vi "player tansition data for all2.vi"() -> ()   [LabVIEW 2013]
panel:
  out "CJ opp ALL":string[][](array[string])
  out "CJ opp left":string[][](array[string])
  out "CJ opp right":string[][](array[string])
  in  "CJ top vs WF":string[][](array[string])=[["3", "36585", "36833", "0 -4 4 -4 0 3 0 4 -4\r\n"], ["3", "37249", "37305", "0 4\r\n"], ["3", "37585", "38105", "1 0 1 -4 1 -4 1 0 2 -2 2 0 -4 0 -2 3 0 -1 1 0 4 -4 1\r\n"], ["3", "38889", "39001", "0 -3 3 0\r\n"], ["3", "39393", "39729", "2 -1 0 4 -1 4 -4 0 -1 1 0 -3 0 -4 1\r\n"], ["3", "40225", "40345", "-4 0 -4 0\r\n"], ["3", "40921", "41041", "-1 0 -1 0 4 0\r\n"], ["3", "41457", "42113", "0 -3 3 0 2 -2 2 0 -3 0 1 0 1 -4 4 -4 1 0 3 -2 0 1 -1 0\r\n"], ["3", "43049", "43241", "0 1 0 2\r\n"], ["3", "43713", "43961", "0 4 -4 1 -4 1 -4 1 -4 0 -3 3 0 2 0 -4\r\n"], ["3", "44425", "44681", "-4 1 0 2 -2 0 -2 3 0 1 0\r\n"], ["3", "45281", "45617", "0 -3 3 0 -1 1 0 -1 0 4 0 -3 4 -4 1 -4 0\r\n"], ["3", "46169", "46585", "0 1 0 3 -3 0 -2 3 -3 0 4 -4 0\r\n"], ["3", "47177", "47593", "0 4 -4 0 -1 0 3 -3 0 -4 0 1 0 -4 4 -4 1\r\n"], ["3", "48425", "49361", "0 1 0 4 -3 0 2 -1 0 4 0 -4 4 -4 0 -4 4 -4 0 4 0 1 0 3 0 -2 3 -2 0 3 -3 0 1 0 4 0 -2\r\n"], ["3", "49961", "50073", "0 1 -1 0\r\n"], ["3", "50529", "50737", "0 -1 0 3 0 -4 4\r\n"], ["3", "52529", "52657", "0 -3 0 -2 2 0 -1 1\r\n"], ["3", "53009", "53137", "0 4 -4 0\r\n"], ["3", "53569", "54641", "0 -3 3 0 3 -3 0 -4 4 -4 0 4 -4 1 0 2 0 -2 3 -2 0 3 0 4 -4 0 2 -2 0 1 -4 4 -4 0 3 0 2 -1 0 1 -4 1 0 3 -2 0 3 0 1\r\n"], ["3", "55161", "55361", "1 0 1 0 2\r\n"], ["3", "55993", "56281", "0 3 -3 0 2 -2 0 3 -2 0 4 -4 1\r\n"], ["3", "57161", "57321", "0 4 -4 0 -1 0 -3 3 0\r\n"], ["3", "57777", "57833", "0\r\n"], ["3", "58105", "58217", "0 4 0 -4\r\n"], ["3", "58521", "58633", "0 -1 2 -1 0 3\r\n"], ["3", "58905", "59305", "0 3 0 -2 2 0 -3 3 -3 0 4 0 3 -2 2 0 -4 4 -4 4 -4\r\n"], ["3", "59665", "60121", "-4 1 -4 1 -4 4 -3 0 3 0 -2 0 4 0 3 0 1 -4 0 -4 4 -4\r\n"], ["3", "60577", "61201", "0 3 0 -4 4 -3 0 -2 0 4 0 3 0 2 0 2 0 4 0 -4 4 -4 0\r\n"], ["3", "61521", "61689", "0 1 0 -4 4 -4 0 -1\r\n"]]
  in  "WF bottom vs CJ":string[][](array[string])=[["3", "36585", "36833", "2 -2 0 4 0 -4 1 -4 0 3 -2\r\n"], ["3", "37249", "37305", "1 0 2\r\n"], ["3", "37585", "38105", "0 3 0 2 -2 3 -3 0 1 0 -3 3 0 4 0 2 -2 2 -2 3 0\r\n"], ["3", "38889", "39001", "2 0 -2 3 2\r\n"], ["3", "39393", "39729", "0 1 0 4 -4 1 -1 2 -2 3 -3 0 -2\r\n"], ["3", "40225", "40345", "0 -3 4 -3 0 2\r\n"], ["3", "40921", "41041", "0 2 -2 3\r\n"], ["3", "41457", "42113", "0 -4 0 -4 1 0 3 0 1 0 2 -2 0 -3 4 0 4 -3 0 3 -3 -2 0 -3 4 0 -4 0 3 0\r\n"], ["3", "43049", "43241", "-2 2 -2 3 -3 0 -4 1\r\n"], ["3", "43713", "43961", "0 -2 0 2 0 4 0\r\n"], ["3", "44425", "44681", "0 -3 0 -4 0 -3 4 0 -2 3 -3\r\n"], ["3", "45281", "45617", "2 0 -2 2 0 4 0 1 0 -2 3\r\n"], ["3", "46169", "46585", "0 4 0 3 -2 3 0 -4 4 0 4 0 3 0 3\r\n"], ["3", "47177", "47593", "2 0 -2 0 4 0 3 -2 2 -2 3 0 -2\r\n"], ["3", "48425", "49361", "1 0 3 -3 0 3 0 3 -2 3 -2 3 0 3 0 -1 0 4 0 -4 1 0 3\r\n"], ["3", "49961", "50073", "2 -2 0 -3 4 -3\r\n"], ["3", "50529", "50737", "0 1 0 3 0 -2 2 -2\r\n"], ["3", "52529", "52657", "1 0\r\n"], ["3", "53009", "53137", "2 0 -2 3 -2 2 0\r\n"], ["3", "53569", "54641", "1 0 -4 4 0 3 -2 3 -2 0 4 -3 0 -3 4 0 -4 1 -4 0 2 -2 0 3 -3 0 1 0 3 0 -2 3 0 4 0 -4 1 0 3 0 -3 4 0 2\r\n"], ["3", "55161", "55361", "0 -3 4 -3 0 1 0\r\n"], ["3", "55993", "56281", "0 3 0 4 0 -4 1 0 -2 0\r\n"], ["3", "57161", "57321", "2 -2 0 -2 0 -4\r\n"], ["3", "57777", "57833", "-1 0\r\n"], ["3", "58105", "58217", "2 0 4\r\n"], ["3", "58521", "58633", "1 0 3 0\r\n"], ["3", "58905", "59305", "2 0 -4 4 0 1 0 3 -2 0 4 0 -4 0 3 0 -2 3\r\n"], ["3", "59665", "60121", "0 2 -2 0 -4 0 -4 4 -3 0 -4 1 0 4 0 -3 3 0\r\n"], ["3", "60577", "61201", "1 0 4 -3 0 2 -2 0 4 0 -3 4 -3 0 -4 0 -3 0 -4 1 0 -2 3 -2 0 1\r\n"], ["3", "61521", "61689", "2 -2 3 0\r\n"]]
  in  "WF top vs CJ":string[][](array[string])=[["3", "432", "664", "2 -1 0 4 0 1 0 3 -2\r\n"], ["3", "928", "1240", "0 3 0 -2 3 -2 0 -2 3 -2 2 -1 0 3 0\r\n"], ["3", "1664", "2056", "1 0 1 0 4 -4 0 3 0 3 -2 0 4 0 3 -2\r\n"], ["3", "2632", "2936", "0 3 -2 0 -1 1 0 2 -2 2 0 -3 4\r\n"], ["3", "3368", "3480", "2 0 4\r\n"], ["3", "3824", "4008", "0 -4 4 -4 0 1 -1 0 4\r\n"], ["3", "4376", "4760", "-1 0 4 -4 0 -4 4 -4 0 2 0 -4 0 -3 3 -2 3 -2 0 -4\r\n"], ["3", "5216", "5800", "2 0 -1 2 -1 0 1 -1 0 3 0 -2 0 3 0 -3 0 -3 0 -4 4 -4 1 -1 2 -1 1 0 3 0\r\n"], ["3", "6496", "6568", "0 3\r\n"], ["3", "6920", "7392", "1 0 -3 0 1 -4 0 2 0 -2 3 0 4 -4 0 -1 0 3 0 1\r\n"], ["3", "8560", "8968", "0 -1 2 0 -3 4 0 -1 0 4 -4 4 -4 0 2 -1 1 0 -3 3 0\r\n"], ["3", "9472", "10000", "0 3 -2 3 0 4 0 1 0 4 0 -4 4 -4 0 -4 4 -4 0 3\r\n"], ["3", "10664", "10864", "2 0 3 0 1 0\r\n"], ["3", "11376", "11720", "1 0 -4 1 -1 0 -2 -1 3 -2 2 -2 0 -3 0 1 -1\r\n"], ["3", "12304", "12400", "2 0 3\r\n"], ["3", "12920", "13216", "-4 1 -1 0 3 0 3 0 1\r\n"], ["3", "13680", "14088", "0 4 0 -4 1 0 1 0 3 0 4 -4 0 -4 4 0\r\n"], ["3", "14600", "14784", "2 0 -4 4 0 -1\r\n"], ["3", "15360", "15448", "0 3 -2 2\r\n"], ["3", "15792", "16320", "0 4 0 1 -4 4 -4 0 2 0 -3 4 0 4 -4 0 3 0 -1 1 -4 4 0 1\r\n"], ["3", "17048", "17816", "0 1 -1 0 -4 0 4 0 1 0 4 0 2 0 -4 4 0 2 0 3 0 4 -4 0 3 0 4 0 -4 4\r\n"], ["3", "19864", "20016", "1 0 -4 4 0 2 -1 0\r\n"], ["3", "20648", "21176", "2 0 4 -4 1 -1 0 4 0 -2 2 0 4 -4 0 1 0 4 0 2\r\n"], ["3", "21680", "21888", "0 4 0 3 -2 0 4\r\n"], ["3", "22304", "22488", "0 3 0 -2 3 0 1 -4\r\n"], ["3", "22960", "23120", "1 -4 1 0 -1 0 3 -2 2 0\r\n"], ["3", "23560", "23656", "2 0 -1 0 3\r\n"], ["3", "24056", "24832", "0 -1 0 2 0 -3 4 -4 0 3 0 1 -1 0 -4 4 -4 0 2 -1 1 0 3 0 4 -4 0 3 0 1 0 3 -2\r\n"], ["3", "25672", "26776", "2 -1 0 3 0 4 -4 0 1 -4 1 -1 0 -4 4 0 -4 0 3 -2 0 4 -4 4 -4 0 2 -2 0 1 0 4 0 3 0 3 -2 3 -3 0 3 0 -3 0 1 -4\r\n"], ["3", "27896", "28256", "1 -1 0 -2 3 -3 0 -4 0 -3 0 3 -2 0 3 -2 2\r\n"], ["3", "28824", "28888", "0 4\r\n"], ["3", "29392", "29648", "2 0 -2 3 0 2 -1 0 -3 0 -2 3\r\n"], ["3", "30144", "31080", "1 0 3 0 3 0 -2 3 -2 0 -2 3 -2 0 3 0 1 -1 0 3 0 3 0 4 -4 0 1 -1 0 3 0 -3 0 -4 4 -4 0 3 0 -1 1 -4 1\r\n"], ["3", "32568", "32656", "0 -1 2 0 3\r\n"], ["3", "33080", "33264", "2 0 3 -2 0\r\n"]]
  in  "CJ bottom vs WF":string[][](array[string])=[["3", "432", "664", "0 2 -2 0 3 -3 0 -4 4\r\n"], ["3", "928", "1240", "-4 0 4 0 4 0 -4 0 -2 2 0 4\r\n"], ["3", "1664", "2056", "0 -3 3 0 3 0 3 -3 0 4 -4 0 -4 0 3 -3 0\r\n"], ["3", "2632", "2936", "2 0 4 0 3 -3 0 1 0\r\n"], ["3", "3368", "3480", "0 4 -3 0\r\n"], ["3", "3824", "4008", "-4 0 3 -2 0 1 0 -2\r\n"], ["3", "4376", "4760", "0 -1 1 0 3 0 4 0 -2\r\n"], ["3", "5216", "5800", "0 4 0 -3 3 0 2 0 4 -4 1 -4 0 -3 3 0 3 0 2 0\r\n"], ["3", "6496", "6568", "0 4\r\n"], ["3", "6920", "7392", "0 3 -3 0 -3 3 0 3 0 -3 4 0 4 -4 0 2\r\n"], ["3", "8560", "8968", "-4 1 0 4 -3 0 3 0 4 -3 0 2 0 4\r\n"], ["3", "9472", "10000", "-2 0 1 -4 0 4 -3 0 2 -2 0 3 0 3 0 -2 2 0 4\r\n"], ["3", "10664", "10864", "0 1 0 -2 0 4 -4 0\r\n"], ["3", "11376", "11720", "0 4 -3 0 -1 1 0 1 0\r\n"], ["3", "12304", "12400", "0 3 -3 0\r\n"], ["3", "12920", "13216", "0 2 -1 0 4 -4 0 3 0 2 -2\r\n"], ["3", "13680", "14088", "-4 1 0 3 0 -3 4 0 2 -2 3 -2 2 -2 0 1\r\n"], ["3", "14600", "14784", "0 3 0 -2 0 -4 0\r\n"], ["3", "15360", "15448", "-2 2 0\r\n"], ["3", "15792", "16320", "-4 1 0 -2 0 3 0 1 0 3 0 3 0 4 0 -2 0 -2 2 -2\r\n"], ["3", "17048", "17816", "-2 0 -3 4 -3 0 2 -2 3 -2 0 -2 2 -2 0 4 -3 0 3 -3 0 1 0 3 -3 0 4 -3 0\r\n"], ["3", "19864", "20016", "0 3 0 -4 0 2\r\n"], ["3", "20648", "21176", "0 -4 0 -2 0 -1 1 0 3 -3 0 1 0 3 0 -2 0 3 0 4 0\r\n"], ["3", "21680", "21888", "-4 0 1 0\r\n"], ["3", "22304", "22488", "2 0 4 0\r\n"], ["3", "22960", "23120", "0 2 0\r\n"], ["3", "23560", "23656", "0 2 0\r\n"], ["3", "24056", "24832", "0 3 0 1 0 3 -3 0 4 0 -2 2 0 -4 0 -1 2 0 -3 4 0 -2 0 3 0 -2 0 -1 1 0\r\n"], ["3", "25672", "26776", "0 2 0 4 0 2 0 3 0 -3 0 2 0 3 0 1 -4 0 -2 0 3 0 4 -3 0 2 -2 0 -2 0 4 0 -4 0 -4 1 0 2 0 4 -4 1 -1 0 2\r\n"], ["3", "27896", "28256", "0 1 -4 0 2 -1 0 3 -3 0 -4 1\r\n"], ["3", "28824", "28888", "0\r\n"], ["3", "29392", "29648", "0 4 -3 0 -1 2 -1 0 4 0\r\n"], ["3", "30144", "31080", "0 4 0 2 0 4 0 4 0 4 -4 0 -2 2 0 3 0 2 0 2 -2 0 -2 3 -2 0 1 0 1 0 2\r\n"], ["3", "32568", "32656", "0\r\n"], ["3", "33080", "33264", "0 2 0 4 0 -2 0 1\r\n"]]
  in  "CJ top vs MOM":string[][](array[string])=[["2", "20073", "20100", ""], ["2", "20448", "20856", "0 2 -1 0 -1 0 -4 4 -4 1 0 1 -4 1 0 -1 1 -4\r\n"], ["2", "21525", "21927", "1 0 -1 0 4 -4 1 -4 1 0 4 -4 -1 0 -1\r\n"], ["2", "22452", "22611", "0 -3 3 0 2 -1 0\r\n"], ["2", "23481", "23691", "0 -1 2 0 -3 -4 1 0 1\r\n"], ["2", "24570", "24945", "2 -1 0 -2 2 0 3 -2 0 -4 4 -4 0 4\r\n"], ["2", "25509", "25761", "0 3 0 -3 0 1 0 -4 4\r\n"], ["2", "26238", "26412", "0 2 -1 0 2 0 4\r\n"], ["2", "26931", "27048", "0 4 -4 0 2\r\n"], ["2", "27495", "27927", "0 1 0 3 0 -1 0 -4 0 1 -4 0 -4 0 3 0 -4\r\n"], ["2", "28380", "28440", "-4 1 -4 1\r\n"], ["2", "28887", "29316", "0 -1 0 4 -4 1 -4 1 0 3 0 3 0 -4 0 -4 0 4 -4 1\r\n"], ["2", "30435", "30618", "0 1 0 1 -4 1 0\r\n"], ["2", "31050", "31302", "0 2 0 -4 0 -1 2 -1 0 4 -4\r\n"], ["2", "31932", "32043", "1 -4 1 0 4\r\n"], ["2", "32874", "32955", "0 3 -2\r\n"], ["2", "33441", "33579", "2 0 -1 0\r\n"], ["2", "35214", "35349", "0 2 0 -2 0\r\n"], ["2", "35655", "35907", "0 4 -4 1 -4 1 0 4 -4 1\r\n"], ["2", "36303", "36528", "0 3 0 -2 2 -2 2 0 4\r\n"], ["2", "36942", "37065", "-3 0 -1 0 -3\r\n"], ["2", "37413", "37983", "0 1 -1 0 1 0 -4 1 0 -4 4 0 2 0 4 0 -3 3 0 4 -4 1 -4 1 0 4\r\n"], ["2", "38463", "38574", "-3 0 4 0\r\n"], ["2", "38997", "39213", "-4 1 0 -1 0 -1 0 -2 0\r\n"], ["2", "39612", "40125", "0 3 0 -1 2 -1 0 4 -4 0 -3 0 -1 1 0 2\r\n"], ["2", "40695", "40848", "0 1 0 1 -4 1 0\r\n"], ["2", "41394", "41457", "0 2 -1\r\n"], ["2", "41964", "42060", "1 -4 1 0 4\r\n"], ["2", "42483", "42588", "0 4 0\r\n"], ["2", "42942", "43017", "0 2 -1 0\r\n"], ["2", "43305", "43605", "0 3 -2 0 4 0 4 -4 0 2 0\r\n"]]
  in  "MOM bottom vs CJ":string[][](array[string])=[["2", "20073", "20100", ""], ["2", "20448", "20856", "0 1 0 4 0 3 0 -2 0 3 0 4 0 2 -2 0\r\n"], ["2", "21525", "21927", "0 3 -2 0 4 0 -2 2 -2 0 -2 0 4 0 -2 0 2\r\n"], ["2", "22452", "22611", "2 0 1 -1 0\r\n"], ["2", "23481", "23691", "1 0 -3 4 -3 0 -2 0 3 0\r\n"], ["2", "24570", "24945", "0 3 -2 0 4 0 -3 3 0 3 -2 0\r\n"], ["2", "25509", "25761", "2 0 3 0 1 0 3\r\n"], ["2", "26238", "26412", "1 0 3 -3 0 4 -3 0\r\n"], ["2", "26931", "27048", "-2 2 -2 0\r\n"], ["2", "27495", "27927", "0 1 0 -3 4 0 3 -2 3 0 1 0 4 0 -1\r\n"], ["2", "28380", "28440", "0 3\r\n"], ["2", "28887", "29316", "-2 2 0 3 0 -2 0 2 0 -2 0 3 0 -4 0 -2\r\n"], ["2", "30435", "30618", "0 3 0 -3 4\r\n"], ["2", "31050", "31302", "0 3 -2 2 -2 3 -2 0\r\n"], ["2", "31932", "32043", "-1 0 3 0 3\r\n"], ["2", "32874", "32955", "2 0\r\n"], ["2", "33441", "33579", "0 -3 0 1\r\n"], ["2", "35214", "35349", "1 0 4 -4 1\r\n"], ["2", "35655", "35907", "-2 2 0 4 0 -2 0 -2\r\n"], ["2", "36303", "36528", "1 0 4 0 1 0 -3 3\r\n"], ["2", "36942", "37065", "-2 2 0 3 -2\r\n"], ["2", "37413", "37983", "1 0 -3 4 -3 0 3 0 3 0 -2 0 3 -2 0 1 -4 0 3 0 -2 0 3 -3 0\r\n"], ["2", "38463", "38574", "-2 2 0 2 0 3\r\n"], ["2", "38997", "39213", "0 3 -2 0 3 0 -4 1\r\n"], ["2", "39612", "40125", "0 1 0 -4 4 0 -2 0 3 0 -4 0 4 0 -4 1 0 3 -2 3 0 -1 1 -1\r\n"], ["2", "40695", "40848", "2 0 -3 4 -3 0 2 0\r\n"], ["2", "41394", "41457", "0 3\r\n"], ["2", "41964", "42060", "0 3\r\n"], ["2", "42483", "42588", "-1 0 4\r\n"], ["2", "42942", "43017", "0 3\r\n"], ["2", "43305", "43605", "-2 3 0 1 -4 0 -2 2 -2 3 0 4\r\n"]]
  in  "MOM top vs CJ":string[][](array[string])=[["2", "129", "315", "-2 2 -1 0 1 -4 0 3 -2\r\n"], ["2", "789", "1425", "1 -1 0 4 0 2 -2 3 0 1 -4 1 0 -3 4 0 3 0 4 0 4 0 -4 0\r\n"], ["2", "2196", "2283", "-1 0 4 -4\r\n"], ["2", "2754", "2940", "-1 0 -1 2 0 2 0\r\n"], ["2", "3372", "3732", "-1 0 3 -2 0 2 -2 3 -2 2 -2 0 -3 4 0 1\r\n"], ["2", "4236", "4572", "-2 2 -1 0 2 0 3 -1 3 -2 2 0 -2 2 -2 0 1 0 2 0\r\n"], ["2", "6177", "6336", "1 -4 1 0 4 -4 0 2 0\r\n"], ["2", "6768", "6849", "2 -2 0\r\n"], ["2", "7200", "7488", "0 4 -4 -1 0 -1 1 -1 0 4 0 -2 3 -2 0\r\n"], ["2", "8115", "8613", "-1 0 2 -1 0 4 -4 0 -4 0 4 0\r\n"], ["2", "9147", "9234", "0 -3 0\r\n"], ["2", "9762", "10140", "1 0 -1 2 -1 0 3 0 3 -2 3 -2 0 2\r\n"], ["2", "10554", "10791", "2 0 2 0 -2 3 -2 2 -1 0 4 0 2\r\n"], ["2", "11328", "11625", "-1 1 -4 1 0 1 0 -4 4 -4 0 3 -2 2 -1 0 3 0 -1 1\r\n"], ["2", "12237", "12693", "2 0 -1 1 -1 0 3 -2 3 0 2 0 3 -2 0 -4 0 4 -4 0 4 0\r\n"], ["2", "13377", "13542", "0 -1 0 3 0 2 -2\r\n"], ["2", "13953", "14280", "1 -4 1 -1 0 2 0 3 -2 3 -2 3\r\n"], ["2", "14760", "14850", "2 0\r\n"], ["2", "15306", "15429", "-1 0 3 0 3\r\n"], ["2", "15720", "15909", "1 -4 1 0 -4 4 -4 0\r\n"], ["2", "16497", "16572", "-2 2 -1 0\r\n"]]
  in  "CJ bottom vs MOM":string[][](array[string])=[["2", "129", "315", "-1 0 -3 3 0 1 0 4\r\n"], ["2", "789", "1425", "0 1 0 1 0 4 0 -2 2 0 4 0 -2 0 1 0 3 0 3\r\n"], ["2", "2196", "2283", "-4 1 0\r\n"], ["2", "2754", "2940", "2 0 -1 0 4 -3 0 3 0 -2\r\n"], ["2", "3372", "3732", "-4 0 4 0 -4 1 0 -4 0 -4 4 0 3 0\r\n"], ["2", "4236", "4572", "0 3 -3 0 2 -2 0 -4 4 -4 0 -3 3 0\r\n"], ["2", "6177", "6336", "0 -2 2 -2 0 3\r\n"], ["2", "6768", "6849", "0 -4\r\n"], ["2", "7200", "7488", "0 2 -2 0 2 0 -2\r\n"], ["2", "8115", "8613", "-4 1 0 4 0 -2 2 -2 0 -2 3 -2 0 1 0 1 0 3\r\n"], ["2", "9147", "9234", "0 2 0\r\n"], ["2", "9762", "10140", "0 -3 3 -3 0 3 0 1 -4 0 3 0\r\n"], ["2", "10554", "10791", "0 -3 4 0 1 -4\r\n"], ["2", "11328", "11625", "0 3 0 -2 0 2 -1 0 2 -2 0\r\n"], ["2", "12237", "12693", "0 4 -3 0 2 0 4 -3 0 -2 2 -2 0 -2 0 4\r\n"], ["2", "13377", "13542", "-4 0 1\r\n"], ["2", "13953", "14280", "0 -3 0 -3 0 4 0\r\n"], ["2", "14760", "14850", "-1 0 1 0\r\n"], ["2", "15306", "15429", "0\r\n"], ["2", "15720", "15909", "0 3 0 3 -3 0 3 -3\r\n"], ["2", "16497", "16572", "0 -3\r\n"]]
  in  "CJ top vs HY":string[][](array[string])=[["1", "20809", "20913", "0 1 -1 1 -1 1 0\r\n"], ["1", "21225", "21321", "1 0\r\n"], ["1", "21505", "21729", "2 -2 0 3 0 4 0 -1 0 -1\r\n"], ["1", "22065", "22177", "0 4 -4 1\r\n"], ["1", "22697", "23185", "0 4 -4 0 4 0 -4 1 -1 0 -3 3 0 4 -4 0 -1 0 4\r\n"], ["1", "23537", "24017", "-4 0 -3 0 -4 0 2 0 4 0 -2 0 -1 1 0 4 -4\r\n"], ["1", "24521", "24657", "0 -1 1 0\r\n"], ["1", "25345", "25553", "0 4 0 1 -1 0\r\n"], ["1", "25913", "26209", "0 2 -1 0 -4 4 -4 0 -1 1\r\n"], ["1", "26577", "26857", "2 0 2 0 2 0 -3 0 4 -4 1 0\r\n"], ["1", "27193", "27537", "1 0 4 0 2 0 -2 3 -2 0 4 -4 0\r\n"], ["1", "27921", "28169", "0 4 0 2 0 4\r\n"], ["1", "28753", "28841", "-1 1 -1 2\r\n"], ["1", "29201", "29617", "0 4 -4 0 -1 2 0 -4 1 -4 4 -4 0 -4 4 -3 0 4 -4 1 0 3\r\n"], ["1", "30201", "30257", "0 -1\r\n"], ["1", "30633", "30737", "2 0 2 0 2\r\n"], ["1", "31017", "31217", "0 3 -2 0 -1 1 -1 0 -3 0\r\n"], ["1", "31617", "31713", "2 0\r\n"], ["1", "32225", "32289", "0 3\r\n"], ["1", "33385", "33721", "0 4 -4 1 0 3 -2 2 -2 2 0 4 0 4 0\r\n"], ["1", "34417", "34737", "-4 0 -2 0 2 0 4 -4 1 -4 1 0 1\r\n"], ["1", "35081", "35137", "0\r\n"], ["1", "35449", "35497", "0\r\n"], ["1", "35761", "35833", "0 4\r\n"], ["1", "36129", "36673", "-2 2 0 -1 0 4 -4 1 0 1 -1 0 1 0 4 0 -4 4 0 2 0\r\n"], ["1", "37233", "37313", "0 -1\r\n"], ["1", "37633", "37913", "1 0 4 0 -2 0 -2 0 1\r\n"], ["1", "38409", "38665", "2 0 -4 0 4 -3 0 1\r\n"], ["1", "39097", "39289", "0 -1 1 0 -4 0\r\n"], ["1", "39593", "39729", "-4 1 0 -4 0 -1 1\r\n"], ["1", "39977", "40089", "0 4 0 2\r\n"], ["1", "40441", "40553", "0 3 2 3\r\n"], ["1", "40705", "41337", "2 0 -4 1 -4 4 -3 0 2 -1 1 -1 0 4 0 -3 0 2 0 3 -2 2 0 3\r\n"], ["1", "41745", "41889", "0 1\r\n"]]
  in  "HY bottom vs CJ":string[][](array[string])=[["1", "20809", "20913", "-2 2 -2 0 -1\r\n"], ["1", "21225", "21321", "0 4 -3 0\r\n"], ["1", "21505", "21729", "0 1 0 -1 1\r\n"], ["1", "22065", "22177", "-4 0\r\n"], ["1", "22697", "23185", "-2 0 3 0 1 0 3 -2 0 -1 0 4 0 3 0 -3 3 -3\r\n"], ["1", "23537", "24017", "0 4 0 -2 0 1 0 -4 4 -3 0 1 0 4 0 -4 1 0 3 -3 0\r\n"], ["1", "24521", "24657", "0 -1 2\r\n"], ["1", "25345", "25553", "2 0 -3 4 0\r\n"], ["1", "25913", "26209", "-4 0 -3 3 -3 0 -3 3 0 -2 3 0\r\n"], ["1", "26577", "26857", "0 -1 1 -4 4 -3 0 3 0\r\n"], ["1", "27193", "27537", "0 -1 2 0 3 0 1 -4 4 0 2 0\r\n"], ["1", "27921", "28169", "2 -2 0 -4 0 -4 4 0 -4\r\n"], ["1", "28753", "28841", "1 -1 2 -1\r\n"], ["1", "29201", "29617", "2 0 -2 0 4 0 2 0 3 0 -2 0 -4\r\n"], ["1", "30201", "30257", "1 -1 0 -1\r\n"], ["1", "30633", "30737", "0 1 -4 1\r\n"], ["1", "31017", "31217", "0 4 0 -1 1 -1 0\r\n"], ["1", "31617", "31713", "0 3\r\n"], ["1", "32225", "32289", "-2 0\r\n"], ["1", "33385", "33721", "1 -4 0 -2 0 4 0 -4 0 4 -3 0 1 -4 0 1\r\n"], ["1", "34417", "34737", "0 -3 3 -2 0 3 0 -2 2\r\n"], ["1", "35081", "35137", "1 0\r\n"], ["1", "35449", "35497", "2\r\n"], ["1", "35761", "35833", "0 -4\r\n"], ["1", "36129", "36673", "0 4 0 -4 0 -3 3 -3 0 -2 0 -2 0 4 0 -1 1 0 3 0 -4 1 -4 0 4\r\n"], ["1", "37233", "37313", "2 0 -1 1\r\n"], ["1", "37633", "37913", "0 2 0 4 0 4 -4 0 -1 2\r\n"], ["1", "38409", "38665", "0 3 -2 0 3 -2\r\n"], ["1", "39097", "39289", "1 0 -3 3 0 -4\r\n"], ["1", "39593", "39729", "0 -3 3 0 -1 0\r\n"], ["1", "39977", "40089", "2 -2 0 1\r\n"], ["1", "40441", "40553", "-4 1 -4 1 -4 0\r\n"], ["1", "40705", "41337", "0 4 0 2 0 -4 1 2 -1 0 4 0 1 0 4 -4 4 0 -4 4 0\r\n"], ["1", "41745", "41889", "-2 0 3 0 -2 0\r\n"]]
  in  "HY top vs CJ":string[][](array[string])=[["1", "400", "872", "0 4 0 4 0 4 0 4 0 -2 3 0 3 0 4 0\r\n"], ["1", "1216", "1280", "-4 -1\r\n"], ["1", "1504", "1664", "-2 0 1 0 -4 4\r\n"], ["1", "2584", "2648", "0 4\r\n"], ["1", "2944", "3128", "-2 2 0 -1 -4 1 0 3 0\r\n"], ["1", "3440", "3512", "-1 0 -1 2\r\n"], ["1", "3752", "4232", "0 -1 1 0 4 0 3 -2 0 -2 3 -2 0 4 0 -2 2\r\n"], ["1", "4696", "4816", "2 -1 0 4\r\n"], ["1", "5392", "5624", "0 4 0 2 0 -2 0\r\n"], ["1", "6008", "6296", "1 -1 0 3 0 -4 4 -4 0\r\n"], ["1", "6736", "7016", "2 -1 0 3 -2 0 -3 0 3 0 -3 0\r\n"], ["1", "7344", "7864", "0 4 0 4 -4 1 -1 0 -3 0 1 -4 1 0 4 0 -4 0 -4 4 -4 1\r\n"], ["1", "8368", "8464", "0 -4 1 0 -4 4\r\n"], ["1", "8864", "8992", "0 4 0 -2 2 -2 2 -2 2\r\n"], ["1", "9320", "9704", "-2 2 -1 0 4 0 2 0 4 0 2 -2 0 4\r\n"], ["1", "11288", "11432", "1 0 -1 0 -1 0 1 -1\r\n"], ["1", "11768", "11872", "-2 2 -2 3\r\n"], ["1", "12256", "12536", "1 0 -1 0 -1 2 0 2 -2 0 -4 0\r\n"], ["1", "12888", "13024", "-2 2 0 3 -2 2\r\n"], ["1", "13520", "13632", "0\r\n"], ["1", "13856", "14000", "1 -1 0 3\r\n"], ["1", "14208", "14304", "0 4 0\r\n"], ["1", "14600", "14792", "-2 0 1 -4 0 -3 0\r\n"], ["1", "15280", "15416", "1 0 -1 2 -1 1 -4\r\n"], ["1", "15648", "15760", "0 4\r\n"], ["1", "16672", "16800", "-2 0 -1 1\r\n"], ["1", "17008", "17224", "0 3 0 3 0 3 -2\r\n"], ["1", "17536", "17664", "-4 0 -4 4\r\n"], ["1", "17936", "18144", "0 4 0 -4 0 -4\r\n"], ["1", "18392", "18568", "-2 2 0 4 -4 0 2 -2\r\n"]]
  in  "CJ bottom vs HY":string[][](array[string])=[["1", "400", "872", "2 0 3 -3 0 3 -3 0 4 0 4 0 -2 0 3\r\n"], ["1", "1216", "1280", "0 -1\r\n"], ["1", "1504", "1664", "0 4 0 3 0\r\n"], ["1", "2584", "2648", "-4 0\r\n"], ["1", "2944", "3128", "0 3 0 2 0\r\n"], ["1", "3440", "3512", "0 1\r\n"], ["1", "3752", "4232", "-2 0 -3 3 -2 0 3 -3 0 -4 4 0 1 0 -2 3 0 -3 4 0 1\r\n"], ["1", "4696", "4816", "0 -1 2 0\r\n"], ["1", "5392", "5624", "-4 0 4 -4 0 -2\r\n"], ["1", "6008", "6296", "0 -1 0 4 -3 0 2 -2 3\r\n"], ["1", "6736", "7016", "0 3 0 1 0 3 -3 0 1 0 1\r\n"], ["1", "7344", "7864", "2 0 3 0 2 0 -3 4 0 -3 4 0 2 0 3 0 2\r\n"], ["1", "8368", "8464", "0 3 0\r\n"], ["1", "8864", "8992", "-4 0 2\r\n"], ["1", "9320", "9704", "0 1 0 1 -4 4 -3 0 3 -3 4 0 2 -2\r\n"], ["1", "11288", "11432", "0 4 0 2 -2 0\r\n"], ["1", "11768", "11872", "0 4 0\r\n"], ["1", "12256", "12536", "0 1 -4 4 -4 0 -3 3 0 -2 3\r\n"], ["1", "12888", "13024", "0 1 -4 0 -4\r\n"], ["1", "13520", "13632", "0 2 0 4\r\n"], ["1", "13856", "14000", "0 -1 0 4\r\n"], ["1", "14208", "14304", "-4 0 -2 3\r\n"], ["1", "14600", "14792", "0 3 0 1 -4 0 -4\r\n"], ["1", "15280", "15416", "0 1 -1 2\r\n"], ["1", "15648", "15760", "0 3 -3 0\r\n"], ["1", "16672", "16800", "0 4 0 -1 2\r\n"], ["1", "17008", "17224", "-4 0 -4 4 0 4 0 -4 4\r\n"], ["1", "17536", "17664", "0 3 -2 0\r\n"], ["1", "17936", "18144", "0 3 -2 3 -2 2\r\n"], ["1", "18392", "18568", "0 1 0 4\r\n"]]
  in  "DU top vs CJ":string[][](array[string])=[["0", "26327", "26487", "0 -1 0 -4 4 -4 1 -4 0\r\n"], ["0", "26887", "27583", "1 -4 1 0 2 0 -3 0 2 0 -2 0 1 0 1 -4 4 -4 1 0 3 -2 0 -4 4 -4\r\n"], ["0", "28239", "28431", "0 1 -4 4 -4 1\r\n"], ["0", "28951", "29255", "0 3 0 -3 3 0 1 0 1 -4 4\r\n"], ["0", "29679", "29807", "0 1 -4 0 1 -4\r\n"], ["0", "30287", "30679", "0 3 -2 0 1 -4 1 0 2 0 4 0 4 0 -1 2 -1 0\r\n"], ["0", "31439", "31615", "1 0 -1 0 2 0 4 -4\r\n"], ["0", "32031", "32071", "-4\r\n"], ["0", "32479", "32535", "-1 0 4\r\n"], ["0", "32895", "33079", "0 1 -1 0 1 -4 0\r\n"], ["0", "33431", "33951", "-1 0 1 -4 0 3 0 2 0 4 0 -4 4 -4 0 -1 0 -4 0 -2 0 4\r\n"], ["0", "34559", "34663", "0 4 0\r\n"], ["0", "35127", "35551", "0 4 -4 0 2 -1 0 2 0 4 -4 1 -4 4 0 3\r\n"], ["0", "36151", "36335", "0 4 0 2 0\r\n"], ["0", "36999", "37287", "1 0 -1 1 0 -4 1 -4 1 0 -4\r\n"], ["0", "37759", "37871", "0 3 -2 0 -4\r\n"], ["0", "38463", "38631", "2 -1 0 -4 4 -4 0 2 0 4\r\n"], ["0", "39079", "39143", "1 0\r\n"], ["0", "39535", "39671", "-1 0 -1 1 0 -4\r\n"], ["0", "40047", "40143", "0 3 0\r\n"], ["0", "40575", "40903", "0 -4 4 -4 0 -4 0 4 0 2 0 1 -4 4\r\n"], ["0", "42623", "42759", "-1 0 1 -4\r\n"], ["0", "43111", "43263", "-1 0 2 -1 0 2\r\n"], ["0", "43639", "43839", "1 -1 0 4 -4 1\r\n"], ["0", "44399", "44591", "-1 0 1 -4 4 -4 0 -4 4\r\n"], ["0", "45071", "45335", "0 3 0 3 0 1 -1 0 1\r\n"], ["0", "45959", "46223", "-1 0 4 0 4 -4 1 0 -4 0\r\n"], ["0", "46759", "46855", "1 0 4\r\n"], ["0", "47431", "47767", "0 -1 0 2 -1 0 -2 3 -2 0 -4 4 -4\r\n"], ["0", "48295", "48415", "0 3 0\r\n"], ["0", "48847", "49079", "2 -1 0 1 -4 4 -4 0 2 0\r\n"], ["0", "49623", "50079", "0 4 -4 1 0 1 0 1 -4 0 2 0 4 0 4 -4 1\r\n"], ["0", "50623", "50823", "1 -1 0 3 0 3 0 1 0 4\r\n"], ["0", "51311", "51479", "0 -4 0 -2 0 -4\r\n"], ["0", "52071", "52263", "0 -4 4 -4 0 -2 0 2 0\r\n"], ["0", "52935", "53047", "-1 0 4 -4 0\r\n"], ["0", "53503", "53647", "1 0 -1 2 0 4\r\n"], ["0", "54031", "54199", "0 2 0 -2 0\r\n"], ["0", "54655", "54935", "0 1 -4 0 -4 0 3 -2 0 -4 0 -4 4 -4 1\r\n"]]
  in  "CJ bottom vs DU":string[][](array[string])=[["0", "26327", "26487", "0 1 0 3 -2 3\r\n"], ["0", "26887", "27583", "0 2 -2 3 -3 0 -3 3 -2 2 0 -4 4 -4 1 0 4 0 2 -2 0 4 0 4 0 2 -2 2\r\n"], ["0", "28239", "28431", "0 -3 3 0 -2\r\n"], ["0", "28951", "29255", "1 0 -2 0 4 0 1 0 -2 2 -2\r\n"], ["0", "29679", "29807", "-2 0 3 0\r\n"], ["0", "30287", "30679", "-4 0 -2 0 3 -3 0 -2 2 -2 0 -4 0 3 -2 0\r\n"], ["0", "31439", "31615", "0 -3 4 0 1 0 -2\r\n"], ["0", "32031", "32071", "-2\r\n"], ["0", "32479", "32535", "-4 0\r\n"], ["0", "32895", "33079", "-2 0 -3 4 -3 4 -4\r\n"], ["0", "33431", "33951", "0 1 -4 0 -2 2 -2 0 -4 0 -3 3 -2 3 0 1 0\r\n"], ["0", "34559", "34663", "0 3\r\n"], ["0", "35127", "35551", "0 2 0 3 0 1 0 -2 2 -2 3 0\r\n"], ["0", "36151", "36335", "-1 0 -1 1 0 4 -4 4 -4\r\n"], ["0", "36999", "37287", "0 -3 4 -3 -2 2 -2 3 -2 2 -2 0\r\n"], ["0", "37759", "37871", "2 0 -3 3\r\n"], ["0", "38463", "38631", "0 3 0 -1 0\r\n"], ["0", "39079", "39143", "0 3\r\n"], ["0", "39535", "39671", "0 3 0 3\r\n"], ["0", "40047", "40143", "-4 0 -4 1 -4\r\n"], ["0", "40575", "40903", "2 -2 0 3 -3 0 1 0 -1 0 4 -3 0 2 -2 0\r\n"], ["0", "42623", "42759", "0 1 0 4 -4 4 0\r\n"], ["0", "43111", "43263", "0 1 0 -3 3 -3 0\r\n"], ["0", "43639", "43839", "0 -3 4 0 -4 1 0 -2\r\n"], ["0", "44399", "44591", "0 3 0 -2\r\n"], ["0", "45071", "45335", "2 0 -3 3 -2 2 0 -2 0 -3 4 -3\r\n"], ["0", "45959", "46223", "0 1 0 3 0\r\n"], ["0", "46759", "46855", "0 3 0 -2\r\n"], ["0", "47431", "47767", "-4 0 3 0 2 -1 0 3 0\r\n"], ["0", "48295", "48415", "2 0 4 0 -2 2\r\n"], ["0", "48847", "49079", "0 -3 4 -3 0 -2 2 -2 0 4\r\n"], ["0", "49623", "50079", "0 3 -2 0 -3 4 0 3 0 1 -1 0 -1 0\r\n"], ["0", "50623", "50823", "0 -3 4 -3 0\r\n"], ["0", "51311", "51479", "2 0 3 -3 0 -4 0 -2\r\n"], ["0", "52071", "52263", "-1 0 3 -3 0 1 0 4\r\n"], ["0", "52935", "53047", "0 1 0\r\n"], ["0", "53503", "53647", "0 -1 0 -1 1 -1 0\r\n"], ["0", "54031", "54199", "0 -3 3 -3 0 1 -4 0 -1 0\r\n"], ["0", "54655", "54935", "2 0 3 -2 0 -2 3 -2 0\r\n"]]
  in  "CJ top vs DU":string[][](array[string])=[["0", "756", "1128", "0 3 0 1 0 -3 0 -3 3 0\r\n"], ["0", "1488", "1548", "1 -4\r\n"], ["0", "1914", "2118", "2 0 2 0 -1 0 -3\r\n"], ["0", "2502", "2568", "0 4\r\n"], ["0", "3078", "3456", "0 -1 2 -1 0 2 0 3 0 1 -4 1 0 -4 4 -4\r\n"], ["0", "3996", "4182", "0 -1 0 -4 0 -2 0\r\n"], ["0", "4806", "4926", "1 -1 1 0 -4\r\n"], ["0", "5326", "5462", "-1 0 -4 0 1 0\r\n"], ["0", "5950", "6022", "0 3\r\n"], ["0", "6566", "6934", "-1 1 0 -4 1 0 -4 0 -1 2 0\r\n"], ["0", "7398", "7494", "1 0 -1 0 2\r\n"], ["0", "8142", "8262", "0 -1 -4 1 0 -3 3\r\n"], ["0", "8590", "8670", "2 -1 0\r\n"], ["0", "9062", "9486", "0 4 0 2 0 -3 0 1 -1 0 1 -4 4 -4 4 -4 0 3\r\n"], ["0", "9998", "10526", "0 -4 4 -4 0 -1 2 0 3 -3 0 -3 3 0 -4 1 0 -3 0 3 -2\r\n"], ["0", "11198", "11310", "0 3 0\r\n"], ["0", "11702", "11894", "0 4 0 1 0 -4 4\r\n"], ["0", "13350", "13486", "0 -1 0 4 0\r\n"], ["0", "13886", "14430", "1 -1 0 4 0 2 -2 0 -4 1 -4 4 -3 0 -4 0 -3 3 0 -4 1 -1 2 -1 0 4\r\n"], ["0", "15494", "16030", "0 3 0 4 -4 4 -4 1 -4 1 -4 4 -4 1 -4 0 -3 3\r\n"], ["0", "16694", "16726", ""], ["0", "17134", "17174", "0\r\n"], ["0", "17582", "17798", "0 4 -4 0 -4 0 4 -4 0\r\n"], ["0", "18334", "18374", "1 -4\r\n"], ["0", "18782", "18846", "0 4\r\n"], ["0", "19214", "19382", "0 1 -4 1 -4 0 -4 4 -4 0\r\n"], ["0", "19766", "19966", "-2 2 0 -3 3 -3 0 3 0\r\n"], ["0", "20406", "20526", "1 0 4 0\r\n"], ["0", "20982", "21118", "0 3 0 1 0\r\n"], ["0", "21590", "21726", "0 4 -4 0 -4 1 -4 0\r\n"], ["0", "22230", "22278", "0\r\n"], ["0", "22598", "22862", "0 -4 4 -4 0 -3 3 -2 0 2\r\n"], ["0", "23278", "23646", "0 3 0 1 0 -4 4 0 -3 3 0 -4 0\r\n"]]
  in  "DU bottom vs CJ":string[][](array[string])=[["0", "756", "1128", "-2 0 3 0 -3 0 4 -4 0\r\n"], ["0", "1488", "1548", "0 3\r\n"], ["0", "1914", "2118", "0 4 -3 0 -4 1 0 4 -3 0\r\n"], ["0", "2502", "2568", "0\r\n"], ["0", "3078", "3456", "-2 0 3 -3 0 -4 1 -4 0 3 -3 4 -3 0 2 0 3\r\n"], ["0", "3996", "4182", "0 3 0 1\r\n"], ["0", "4806", "4926", "0 1 0 3\r\n"], ["0", "5326", "5462", "0 3 -2 0 4\r\n"], ["0", "5950", "6022", "0\r\n"], ["0", "6566", "6934", "0 -3 4 0 2 -2 0 -3 0 3 -2 3 -3 4\r\n"], ["0", "7398", "7494", "0 -3 4 -3 0\r\n"], ["0", "8142", "8262", "-2 0 -2 2 0\r\n"], ["0", "8590", "8670", "0 3 -2\r\n"], ["0", "9062", "9486", "0 4 -3 0 3 -2 0 -3 4 -3 0 3 -2 2 -2 0 4 0\r\n"], ["0", "9998", "10526", "2 0 1 -4 0 3 0 -4 4 0 -4 4 0 2 0 4 0 -3 4 -3 0 -4 0 4\r\n"], ["0", "11198", "11310", "0 4\r\n"], ["0", "11702", "11894", "-2 0 -2 0 3 0\r\n"], ["0", "13350", "13486", "0 3 0 -2 3\r\n"], ["0", "13886", "14430", "0 4 0 4 -4 0 2 0 -4 4 -3 0 -2 2 -2 0 4 -3 0 2 0 3 0\r\n"], ["0", "15494", "16030", "0 4 -3 0 1 -1 0 3 0 -2 2 -2 0 -3 4 -3 0 4 -4 1 0\r\n"], ["0", "16694", "16726", ""], ["0", "17134", "17174", "0 -3\r\n"], ["0", "17582", "17798", "2 0 3 0 1 0 -2 3\r\n"], ["0", "18334", "18374", "0\r\n"], ["0", "18782", "18846", "1 -1 0\r\n"], ["0", "19214", "19382", "0 -2 3 0\r\n"], ["0", "19766", "19966", "0 1 0 4 0 4 -4 4\r\n"], ["0", "20406", "20526", "0 1 -1 0 3\r\n"], ["0", "20982", "21118", "0 2 -2 3 -3 4\r\n"], ["0", "21590", "21726", "-2 2 0 -2 3\r\n"], ["0", "22230", "22278", "0 -1\r\n"], ["0", "22598", "22862", "0 4 -4 4 0 3 0 -2 0 -4 0 1 -4\r\n"], ["0", "23278", "23646", "-2 0 4 0 -3 3 0 -2 2 -2 0 -4 0 4 0\r\n"]]
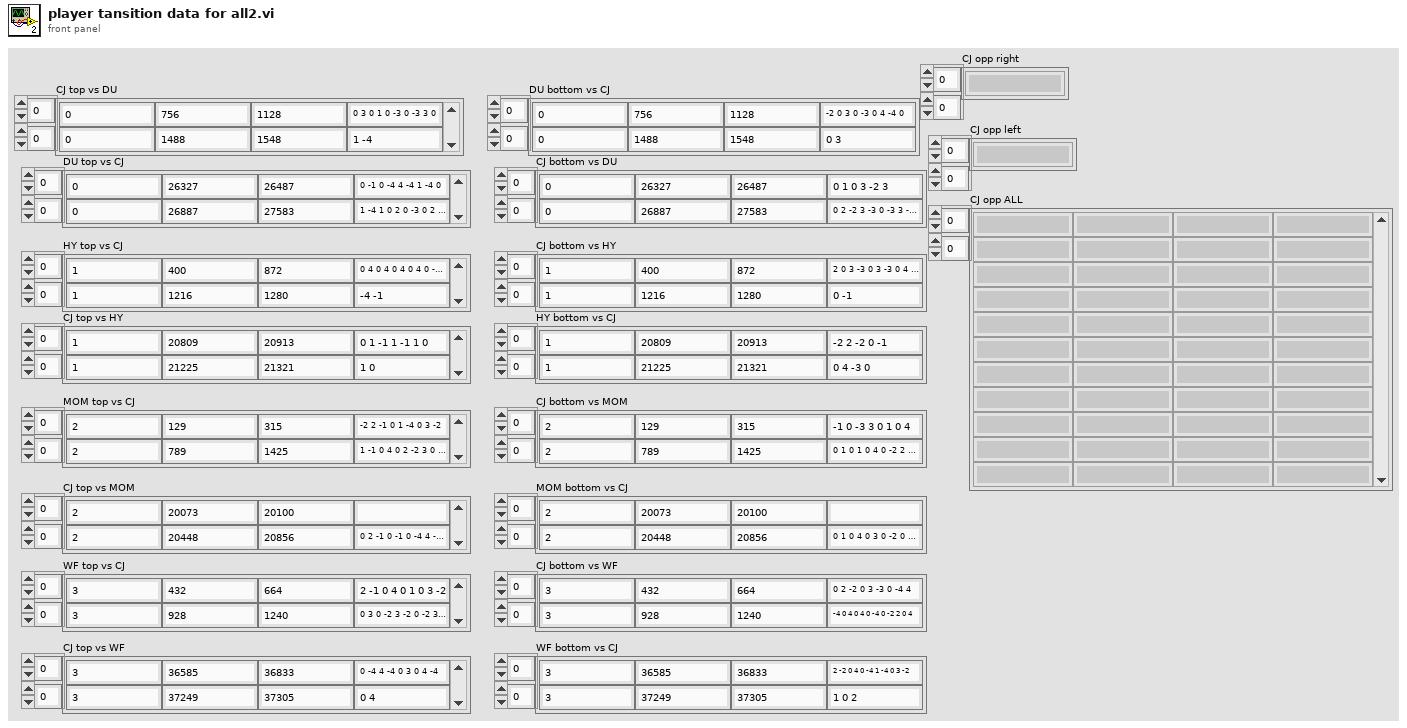
[diagram p1: front panel]
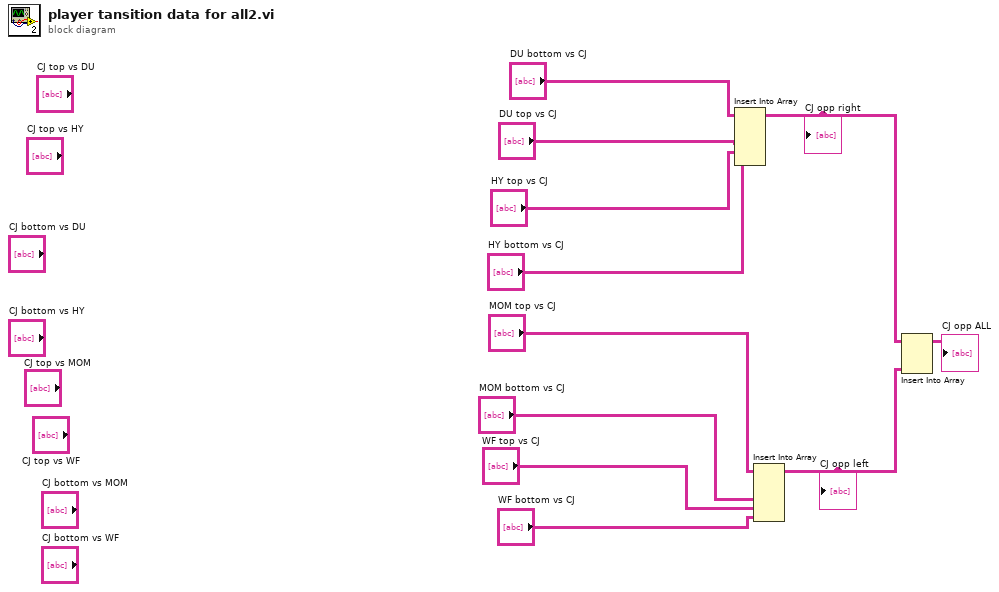
[diagram p0: block diagram]
diagram:
  n1 = Insert Into Array(array="DU bottom vs CJ", new element #1="DU top vs CJ", new element #2="HY top vs CJ", new element #3="HY bottom vs CJ") -> (w3:string[][])  [unwired: 2 in]
  "CJ opp right" <- w3
  n2 = Insert Into Array(array="MOM top vs CJ", new element #1="MOM bottom vs CJ", new element #2="WF top vs CJ", new element #3="WF bottom vs CJ") -> (w2:string[][])  [unwired: 2 in]
  "CJ opp left" <- w2
  n3 = Insert Into Array(array=w3, new element=w2) -> (→"CJ opp ALL":string[][])  [unwired: 2 in]
